vi "practica 2.vi"() -> ()   [LabVIEW 2013]
panel:
  out "Waveform Chart":dbl(graph)
  out "output variable":dbl
  out "alcance":dbl
  out "tiempo":i32
  in  "velocidad inicial":dbl
  in  "cateto adyacente":dbl
  in  "cateto opuesto":dbl
  in  "stop":bool
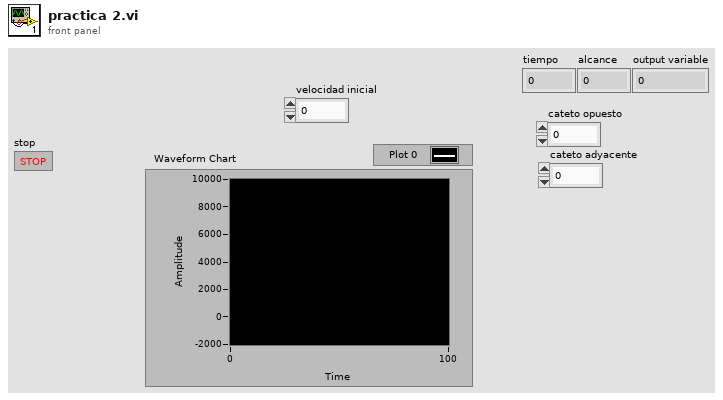
[diagram p1: front panel]
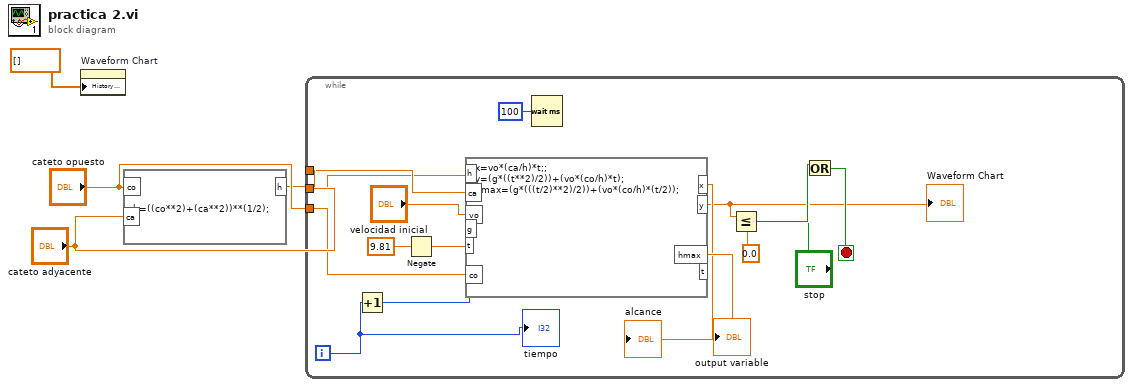
[diagram p0: block diagram]
diagram:
  n1 = property on="Waveform Chart" class="WFChart (strict)"("History Data"=dbl[] []) -> ()  [unwired: 2 in, 2 out]
  n2 = formula code="h=((co**2)+(ca**2))**(1/2);"("co"="cateto opuesto", "ca"="cateto adyacente") -> ("h"=w2:dbl)
  n3 = while {
    tunnel: "cateto opuesto" -> [w16]
    tunnel: "cateto adyacente" -> [w17]
    tunnel: w2 -> [w18]
    i -> [w9]
    stop <- w12 stop-if-true
    n4 = Increment(x=w9) -> (x+1=w11:i32)
    n5 = Negate(x=9.81) -> (-x=w8:dbl)
    n6 = formula code="x=vo*(ca/h)*t;;\ny=(g*((t**2)/2))+(vo*(co/h)*t);\nhmax=(g*(((t/2)**2)/2))+(vo*(co/h)*(t/2));"("t"=w11, "vo"="velocidad inicial", "ca"=w18, "co"=w16, "h"=w17, "g"=w8) -> ("y"=w5:dbl, "hmax"=→"output variable":dbl, "x"=→"alcance":dbl)  [unwired: 1 out]
    "Waveform Chart" <- w5
    n7 = Wait (ms)(milliseconds to wait=u32 100) -> ()  [unwired: 1 out]
    n8 = Less Or Equal?(x=w5, y=0.0) -> (x <= y?=w14:bool)
    n9 = Or(x=w14, y="stop") -> (x .or. y?=w12:bool)
    "tiempo" <- w9
  }
